vi "Begin.vi"   [LabVIEW 2012]
doc: "Called before other user functions, this VI is expected to open initial I/O refnums, load in file data, and do all program initialization. Notice that the <B>error out</B> terminal is simply used for data flow. Wiring it to other structures or subVIs ensures that this VI runs first."
uses:
  <vilib>/Rock Robotics/SystemInterfaces/Typedef/FPGA_TypedefDigitalModule.ctl
  <vilib>/Rock Robotics/SystemInterfaces/DIO/FPGA_DIOPWMChannel.ctl
  <vilib>/Rock Robotics/SystemInterfaces/DIO/FPGA_DIORelayChannel.ctl
  <vilib>/Rock Robotics/WPI/Relay/WPI_RelayDirection.ctl
  <vilib>/Rock Robotics/WPI/Joystick/WPI_JoystickDeviceEnum.ctl
  <vilib>/Rock Robotics/WPI/SafetyOutput/WPI_SafetyOutputConfigMenu.ctl
  <vilib>/Rock Robotics/WPI/MotorControl/WPI_MotorControlOpen Victor.vi
  <vilib>/Rock Robotics/WPI/MotorControl/WPI_MotorControlOpen Jaguar.vi
  <vilib>/Rock Robotics/WPI/RobotDrive/WPI_RobotDriveOpen4MotorWithJaguar.vi
  <vilib>/Rock Robotics/WPI/RobotDrive/WPI_RobotDriveOpen2MotorWithJaguar.vi
types:
  T1 = typedef "WPI_SafetyOutputConfigMenu.ctl" = enum16{"Enable", "Disable"}
  T2 = typedef "FPGA_DIOPWMChannel.ctl" = enum8{"PWM 1", "PWM 2", "PWM 3", "PWM 4", "PWM 5", "PWM 6", "PWM 7", "PWM 8", "PWM 9", "PWM 10", "Invalid"}
  T3 = typedef "WPI_RobotDriveDevRef.ctl" = cluster{"DevStatus":errorcluster, "Motors[]":T4[], "Square Inputs":bool, "Max Output":dbl, "Isochronous":bool}
  T4 = typedef "WPI_MotorControlDeviceRef.ctl" = cluster{"DeviceStatus":errorcluster, "Type":enum16{"PWM", "CAN"}, "PWM":cluster{"Digital Module":T5, "PWM Channel":T2, "DeadBand":T6}, "CAN":cluster{"Device Number":u8, "Control Mode":T7, "Semaphore":T8, "Max Vout":dbl}, "Invert":bool, "TransformRef":T9, "InvTransformRef":T9}
  T5 = typedef "FPGA_TypedefDigitalModule.ctl" = enum16{"Digital Module 1", "Digital Module 2"}
  T6 = typedef "WPI_PWMDeadband.ctl" = cluster{"Name":string, "maxPositivePwm":i32, "minPositivePwm":i32, "centerPwm":i32, "maxNegativePwm":i32, "minNegativePwm":i32, "angularRange":u16}
  T7 = typedef "WPI_CANJaguar_ControlMode.ctl" = enum8{"Percent VBus", "Current", "Speed", "Position", "Voltage"}
  T8 = typedef "Semaphore RefNum" = refnum<k1>
  T9 = typedef "WPI_PWMTransform_ConPane.ctl" = refnum<vi>
  T10 = typedef "WPI_RelayDirection.ctl" = enum16{"Both directions", "Forward only", "Reverse only"}
  T11 = typedef "FPGA_DIORelayChannel.ctl" = enum8{"Relay 1", "Relay 2", "Relay 3", "Relay 4", "Relay 5", "Relay 6", "Relay 7", "Relay 8", "Invalid"}
  T12 = typedef "WPI_ServoDeviceRef.ctl" = cluster{"DeviceStatus":errorcluster, "Digital Module":T5, "PWM Channel":T2, "DeadBand":T6}
  T13 = typedef "WPI_RelayDevRef.ctl" = cluster{"DevStatus":errorcluster, "Relay Channel":T11, "Digital Module":T5, "Relay Direction":T10}
  T14 = typedef "WPI_JoystickDeviceEnum.ctl" = enum16{"USB 1", "USB 2", "USB 3", "USB 4", "Kinect 1", "Kinect 2"}
  T15 = typedef "WPI_JoystickDevRef.ctl" = cluster{"Device":T14}
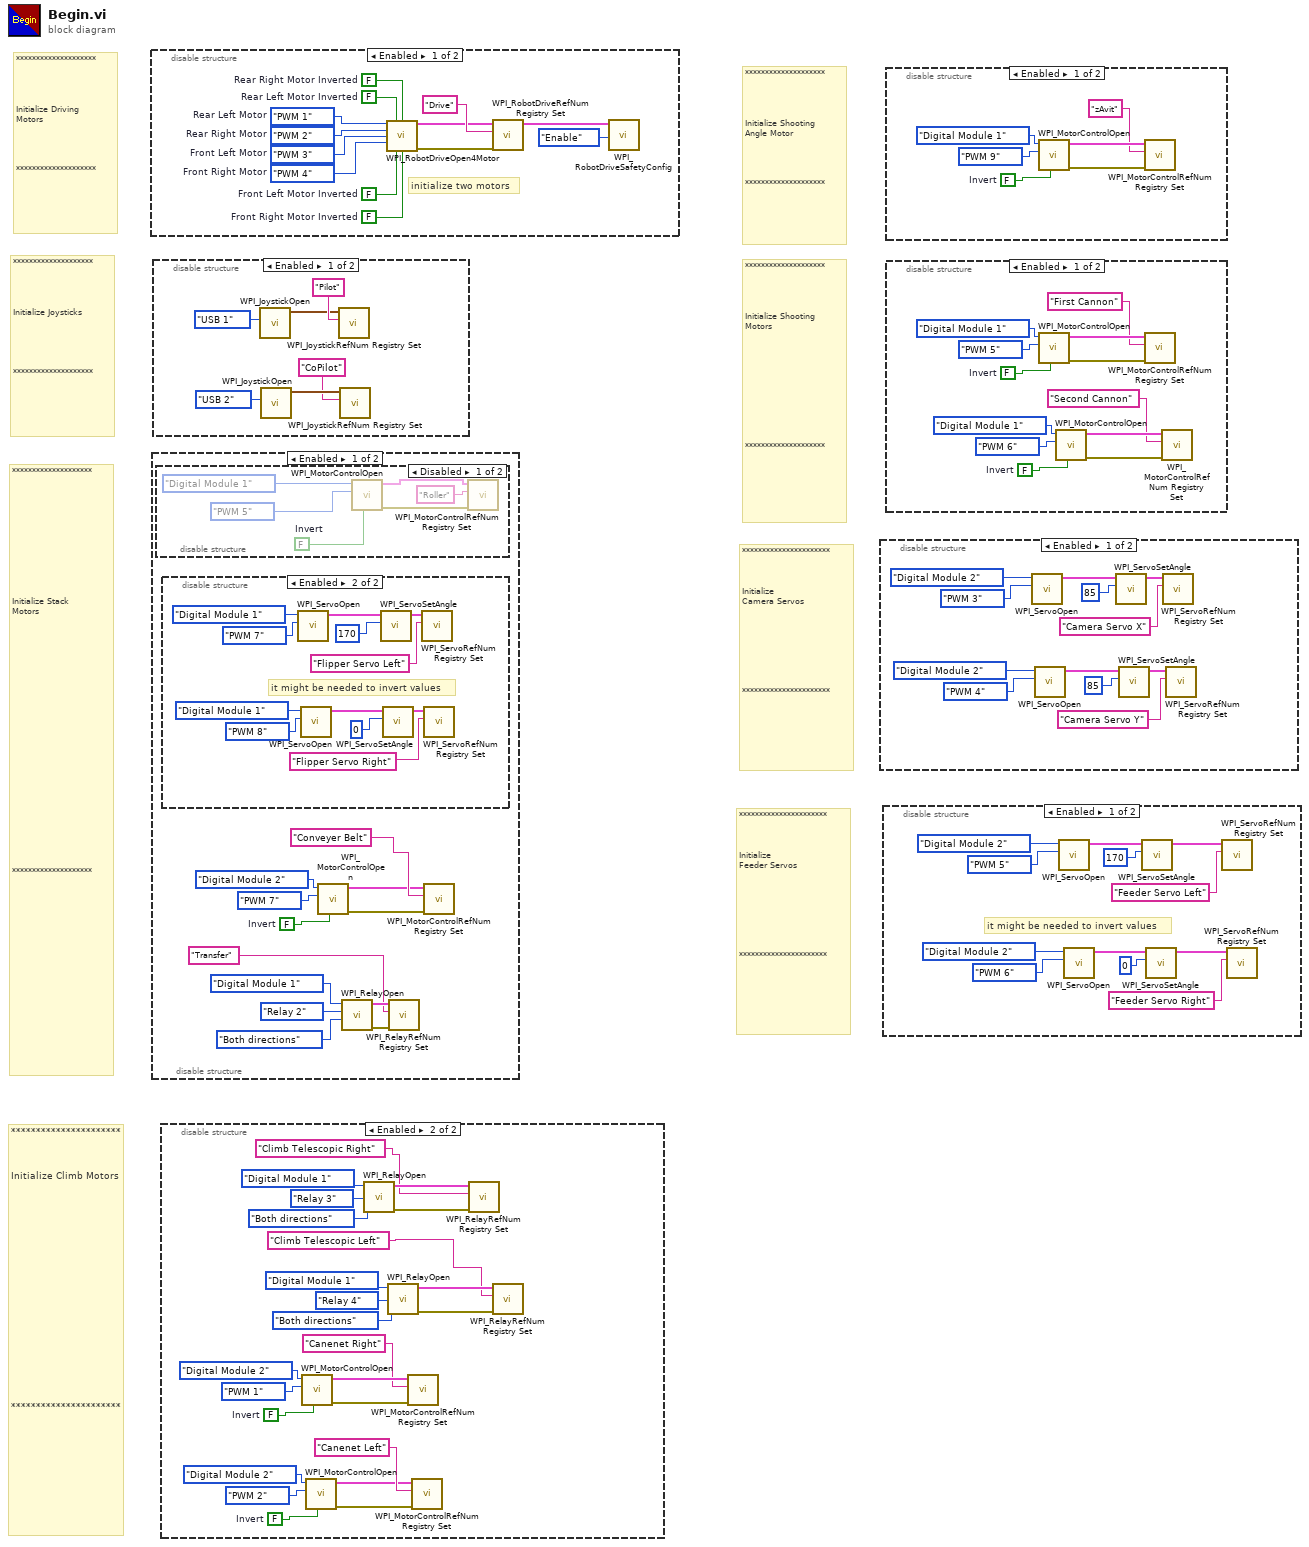
[diagram p0: block diagram]
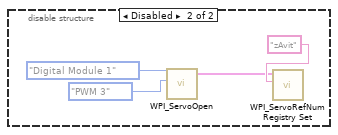
[diagram p5: hidden frame]
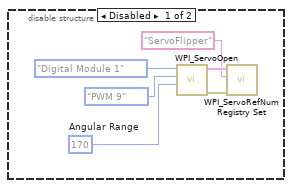
[diagram p9: hidden frame]
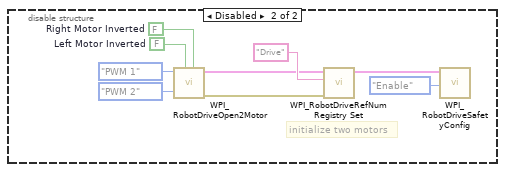
[diagram p11: hidden frame]
diagram:
  # "**********************\n\n\n\nInitialize\nFeeder Servos\n\n\n\n\n\n\n\n\n**********************"
  # "**********************\n\n\n\nInitialize\nCamera Servos\n\n\n\n\n\n\n\n\n**********************"
  # "**********************\n\n\n\nInitialize Climb Motors          \n\n\n\n\n\n\n\n\n\n\n\n\n\n\n\n\n\n\n\n\n**********************"
  # "********************\n\n\n\n\nInitialize Shooting\nAngle Motor\n\n\n\n\n********************"
  # "********************\n\n\n\n\nInitialize Shooting\nMotors\n\n\n\n\n\n\n\n\n\n\n\n********************"
  # "********************\n\n\n\n\n\n\n\n\n\n\n\n\nInitialize Stack \nMotors\n\n\n\n\n\n\n\n\n\n\n\n\n\n\n\n\n\n\n\n\n\n\n\n\n\n********************"
  # "********************\n\n\n\n\nInitialize Driving\nMotors\n\n\n\n\n********************"
  # "********************\n\n\n\n\nInitialize Joysticks\n\n\n\n\n\n********************"
  n1 = disable-structure shown="Enabled" {
    frame Enabled {
      w1 = FPGA_DIOPWMChannel."PWM 4"  # Front Right Motor
      w2 = FPGA_DIOPWMChannel."PWM 3"  # Front Left Motor
      w3 = FPGA_DIOPWMChannel."PWM 2"  # Rear Right Motor
      w4 = FPGA_DIOPWMChannel."PWM 1"  # Rear Left Motor
      w5 = FALSE  # Front Right Motor Inverted
      w6 = FALSE  # Front Left Motor Inverted
      w7 = FALSE  # Rear Right Motor Inverted
      w8 = FALSE  # Rear Left Motor Inverted
      # "initialize two motors"
      n2 = call-poly <vilib>:"WPI_RobotDriveOpen4Motor.vi"("Rear Left Motor"=w4, "Rear Left Motor Inverted"=w8, "Rear Right Motor Inverted"=w7, "Rear Right Motor"=w3, "Front Left Motor"=w2, "Front Right Motor"=w1, "Front Left Motor Inverted"=w6, "Front Right Motor Inverted"=w5) -> ("RobotDriveDevRef"=w10:T3, "error out"=w9:errorcluster)  [unwired: 6 in]
      n3 = call <vilib>:"WPI_RobotDriveRefNum Registry Set.vi"("error in (no error)"=w9, "refnum name"="Drive", "RobotDriveDevRef"=w10) -> ("RobotDriveDevRef"=w12:T3)  [unwired: 8 out]
      n4 = call <vilib>:"WPI_RobotDriveSafetyConfig.vi"("mode"=WPI_SafetyOutputConfigMenu."Enable", "RobotDriveDevRef"=w12) -> ()  [unwired: 8 in, 2 out]
    }
    frame Disabled {
      w14 = FALSE  # Right Motor Inverted
      w15 = FALSE  # Left Motor Inverted
      # "initialize two motors"
      n5 = call-poly <vilib>:"WPI_RobotDriveOpen2Motor.vi"("Right Motor Inverted"=w14, "Left Motor Inverted"=w15, "Right Motor"=FPGA_DIOPWMChannel."PWM 2", "Left Motor"=FPGA_DIOPWMChannel."PWM 1") -> ("error out"=w18:errorcluster, "RobotDriveDevRef"=w19:T3)  [unwired: 6 in]
      n6 = call <vilib>:"WPI_RobotDriveRefNum Registry Set.vi"("error in (no error)"=w18, "refnum name"="Drive", "RobotDriveDevRef"=w19) -> ("RobotDriveDevRef"=w21:T3)  [unwired: 8 out]
      n7 = call <vilib>:"WPI_RobotDriveSafetyConfig.vi"("mode"=WPI_SafetyOutputConfigMenu."Enable", "RobotDriveDevRef"=w21) -> ()  [unwired: 8 in, 2 out]
    }
  }
  n8 = disable-structure shown="Enabled" {
    frame Enabled {
      w24 = FALSE  # Invert
      n9 = disable-structure shown="Disabled" {
        frame Disabled {
          w36 = FALSE  # Invert
          n10 = call-poly <vilib>:"WPI_MotorControlOpen.vi"("Invert"=w36, "PWM Channel"=FPGA_DIOPWMChannel."PWM 5", "Digital Module (Module 1)"=FPGA_TypedefDigitalModule."Digital Module 1") -> ("error out"=w35:errorcluster, "MotorControlDeviceRef"=w40:T4)  [unwired: 7 in]
          n11 = call <vilib>:"WPI_MotorControlRefNum Registry Set.vi"("error in (no error)"=w35, "refnum name"="Roller", "MotorControlDevRef"=w40) -> ()  [unwired: 7 in, 2 out]
        }
        frame Enabled {
        }
      }
      n12 = disable-structure shown="Enabled" {
        frame Disabled {
          w43 = u16 170  # Angular Range
          n13 = call <vilib>:"WPI_ServoOpen.vi"("Angular Range"=w43, "PWM Channel"=FPGA_DIOPWMChannel."PWM 9", "Digital Module (Module 1)"=FPGA_TypedefDigitalModule."Digital Module 1") -> ("error out"=w42:errorcluster, "ServoDeviceRef"=w46:T12)  [unwired: 7 in]
          n14 = call <vilib>:"WPI_ServoRefNum Registry Set.vi"("error in (no error)"=w42, "refnum name"="ServoFlipper", "ServoDeviceRef"=w46) -> ()  [unwired: 7 in, 2 out]
        }
        frame Enabled {
          # "it might be needed to invert values"
          n15 = call <vilib>:"WPI_ServoOpen.vi"("PWM Channel"=FPGA_DIOPWMChannel."PWM 7", "Digital Module (Module 1)"=FPGA_TypedefDigitalModule."Digital Module 1") -> ("ServoDeviceRef"=w58:T12)  [unwired: 8 in, 1 out]
          n16 = call <vilib>:"WPI_ServoOpen.vi"("PWM Channel"=FPGA_DIOPWMChannel."PWM 8", "Digital Module (Module 1)"=FPGA_TypedefDigitalModule."Digital Module 1") -> ("ServoDeviceRef"=w48:T12)  [unwired: 8 in, 1 out]
          n17 = call <vilib>:"WPI_ServoSetAngle.vi"("Angle"=170, "ServoDeviceRef"=w58) -> ("ServoDeviceRef"=w54:T12)  [unwired: 8 in, 1 out]
          n18 = call <vilib>:"WPI_ServoSetAngle.vi"("Angle"=0, "ServoDeviceRef"=w48) -> ("ServoDeviceRef"=w51:T12)  [unwired: 8 in, 1 out]
          n19 = call <vilib>:"WPI_ServoRefNum Registry Set.vi"("refnum name"="Flipper Servo Left", "ServoDeviceRef"=w54) -> ()  [unwired: 8 in, 2 out]
          n20 = call <vilib>:"WPI_ServoRefNum Registry Set.vi"("refnum name"="Flipper Servo Right", "ServoDeviceRef"=w51) -> ()  [unwired: 8 in, 2 out]
        }
      }
      n21 = call-poly <vilib>:"WPI_MotorControlOpen.vi"("Invert"=w24, "PWM Channel"=FPGA_DIOPWMChannel."PWM 7", "Digital Module (Module 1)"=FPGA_TypedefDigitalModule."Digital Module 2") -> ("error out"=w23:errorcluster, "MotorControlDeviceRef"=w27:T4)  [unwired: 7 in]
      n22 = call <vilib>:"WPI_RelayOpen.vi"("Relay Direction"=WPI_RelayDirection."Both directions", "Relay Channel"=FPGA_DIORelayChannel."Relay 2", "Digital Module (Module 1)"=FPGA_TypedefDigitalModule."Digital Module 1") -> ("error out"=w31:errorcluster, "RelayDevRef"=w30:T13)  [unwired: 7 in]
      n23 = call <vilib>:"WPI_RelayRefNum Registry Set.vi"("error in (no error)"=w31, "refnum name"="Transfer", "RelayDevRef"=w30) -> ()  [unwired: 7 in, 2 out]
      n24 = call <vilib>:"WPI_MotorControlRefNum Registry Set.vi"("error in (no error)"=w23, "refnum name"="Conveyer Belt", "MotorControlDevRef"=w27) -> ()  [unwired: 7 in, 2 out]
    }
    frame Disabled {
    }
  }
  n25 = disable-structure shown="Enabled" {
    frame Enabled {
      n26 = call <vilib>:"WPI_JoystickOpen.vi"("JoystickDevice"=WPI_JoystickDeviceEnum."USB 1") -> ("JoystickDevRef"=w63:T15)  [unwired: 10 in]
      n27 = call <vilib>:"WPI_JoystickOpen.vi"("JoystickDevice"=WPI_JoystickDeviceEnum."USB 2") -> ("JoystickDevRef"=w60:T15)  [unwired: 10 in]
      n28 = call <vilib>:"WPI_JoystickRefNum Registry Set.vi"("refnum name"="Pilot", "JoystickDevRef"=w63) -> ()  [unwired: 8 in, 2 out]
      n29 = call <vilib>:"WPI_JoystickRefNum Registry Set.vi"("refnum name"="CoPilot", "JoystickDevRef"=w60) -> ()  [unwired: 8 in, 2 out]
    }
    frame Disabled {
    }
  }
  n30 = disable-structure shown="Enabled" {
    frame Disabled {
    }
    frame Enabled {
      w81 = FALSE  # Invert
      w84 = FALSE  # Invert
      n31 = call-poly <vilib>:"WPI_MotorControlOpen.vi"("Invert"=w84, "PWM Channel"=FPGA_DIOPWMChannel."PWM 1", "Digital Module (Module 1)"=FPGA_TypedefDigitalModule."Digital Module 2") -> ("error out"=w83:errorcluster, "MotorControlDeviceRef"=w88:T4)  [unwired: 7 in]
      n32 = call-poly <vilib>:"WPI_MotorControlOpen.vi"("Invert"=w81, "PWM Channel"=FPGA_DIOPWMChannel."PWM 2", "Digital Module (Module 1)"=FPGA_TypedefDigitalModule."Digital Module 2") -> ("error out"=w82:errorcluster, "MotorControlDeviceRef"=w77:T4)  [unwired: 7 in]
      n33 = call <vilib>:"WPI_RelayOpen.vi"("Relay Direction"=WPI_RelayDirection."Both directions", "Relay Channel"=FPGA_DIORelayChannel."Relay 3", "Digital Module (Module 1)"=FPGA_TypedefDigitalModule."Digital Module 1") -> ("error out"=w75:errorcluster, "RelayDevRef"=w76:T13)  [unwired: 7 in]
      n34 = call <vilib>:"WPI_RelayOpen.vi"("Relay Direction"=WPI_RelayDirection."Both directions", "Relay Channel"=FPGA_DIORelayChannel."Relay 4", "Digital Module (Module 1)"=FPGA_TypedefDigitalModule."Digital Module 1") -> ("error out"=w69:errorcluster, "RelayDevRef"=w70:T13)  [unwired: 7 in]
      n35 = call <vilib>:"WPI_MotorControlRefNum Registry Set.vi"("error in (no error)"=w83, "refnum name"="Canenet Right", "MotorControlDevRef"=w88) -> ()  [unwired: 7 in, 2 out]
      n36 = call <vilib>:"WPI_MotorControlRefNum Registry Set.vi"("error in (no error)"=w82, "refnum name"="Canenet Left", "MotorControlDevRef"=w77) -> ()  [unwired: 7 in, 2 out]
      n37 = call <vilib>:"WPI_RelayRefNum Registry Set.vi"("error in (no error)"=w75, "refnum name"="Climb Telescopic Right", "RelayDevRef"=w76) -> ()  [unwired: 7 in, 2 out]
      n38 = call <vilib>:"WPI_RelayRefNum Registry Set.vi"("error in (no error)"=w69, "refnum name"="Climb Telescopic Left", "RelayDevRef"=w70) -> ()  [unwired: 7 in, 2 out]
    }
  }
  n39 = disable-structure shown="Enabled" {
    frame Enabled {
      n40 = call <vilib>:"WPI_ServoOpen.vi"("PWM Channel"=FPGA_DIOPWMChannel."PWM 3", "Digital Module (Module 1)"=FPGA_TypedefDigitalModule."Digital Module 2") -> ("ServoDeviceRef"=w97:T12)  [unwired: 8 in, 1 out]
      n41 = call <vilib>:"WPI_ServoOpen.vi"("PWM Channel"=FPGA_DIOPWMChannel."PWM 4", "Digital Module (Module 1)"=FPGA_TypedefDigitalModule."Digital Module 2") -> ("ServoDeviceRef"=w92:T12)  [unwired: 8 in, 1 out]
      n42 = call <vilib>:"WPI_ServoSetAngle.vi"("Angle"=85, "ServoDeviceRef"=w97) -> ("ServoDeviceRef"=w96:T12)  [unwired: 8 in, 1 out]
      n43 = call <vilib>:"WPI_ServoSetAngle.vi"("Angle"=85, "ServoDeviceRef"=w92) -> ("ServoDeviceRef"=w93:T12)  [unwired: 8 in, 1 out]
      n44 = call <vilib>:"WPI_ServoRefNum Registry Set.vi"("refnum name"="Camera Servo X", "ServoDeviceRef"=w96) -> ()  [unwired: 8 in, 2 out]
      n45 = call <vilib>:"WPI_ServoRefNum Registry Set.vi"("refnum name"="Camera Servo Y", "ServoDeviceRef"=w93) -> ()  [unwired: 8 in, 2 out]
    }
    frame Disabled {
    }
  }
  n46 = disable-structure shown="Enabled" {
    frame Enabled {
      # "it might be needed to invert values"
      n47 = call <vilib>:"WPI_ServoOpen.vi"("PWM Channel"=FPGA_DIOPWMChannel."PWM 5", "Digital Module (Module 1)"=FPGA_TypedefDigitalModule."Digital Module 2") -> ("ServoDeviceRef"=w109:T12)  [unwired: 8 in, 1 out]
      n48 = call <vilib>:"WPI_ServoOpen.vi"("PWM Channel"=FPGA_DIOPWMChannel."PWM 6", "Digital Module (Module 1)"=FPGA_TypedefDigitalModule."Digital Module 2") -> ("ServoDeviceRef"=w108:T12)  [unwired: 8 in, 1 out]
      n49 = call <vilib>:"WPI_ServoSetAngle.vi"("Angle"=170, "ServoDeviceRef"=w109) -> ("ServoDeviceRef"=w104:T12)  [unwired: 8 in, 1 out]
      n50 = call <vilib>:"WPI_ServoSetAngle.vi"("Angle"=0, "ServoDeviceRef"=w108) -> ("ServoDeviceRef"=w103:T12)  [unwired: 8 in, 1 out]
      n51 = call <vilib>:"WPI_ServoRefNum Registry Set.vi"("refnum name"="Feeder Servo Left", "ServoDeviceRef"=w104) -> ()  [unwired: 8 in, 2 out]
      n52 = call <vilib>:"WPI_ServoRefNum Registry Set.vi"("refnum name"="Feeder Servo Right", "ServoDeviceRef"=w103) -> ()  [unwired: 8 in, 2 out]
    }
    frame Disabled {
    }
  }
  n53 = disable-structure shown="Enabled" {
    frame Enabled {
      w114 = FALSE  # Invert
      n54 = call-poly <vilib>:"WPI_MotorControlOpen.vi"("Invert"=w114, "PWM Channel"=FPGA_DIOPWMChannel."PWM 9", "Digital Module (Module 1)"=FPGA_TypedefDigitalModule."Digital Module 1") -> ("error out"=w113:errorcluster, "MotorControlDeviceRef"=w118:T4)  [unwired: 7 in]
      n55 = call <vilib>:"WPI_MotorControlRefNum Registry Set.vi"("error in (no error)"=w113, "refnum name"="zAvit", "MotorControlDevRef"=w118) -> ()  [unwired: 7 in, 2 out]
    }
    frame Disabled {
      n56 = call <vilib>:"WPI_ServoOpen.vi"("PWM Channel"=FPGA_DIOPWMChannel."PWM 3", "Digital Module (Module 1)"=FPGA_TypedefDigitalModule."Digital Module 1") -> ("ServoDeviceRef"=w119:T12)  [unwired: 8 in, 1 out]
      n57 = call <vilib>:"WPI_ServoRefNum Registry Set.vi"("refnum name"="zAvit", "ServoDeviceRef"=w119) -> ()  [unwired: 8 in, 2 out]
    }
  }
  n58 = disable-structure shown="Enabled" {
    frame Enabled {
      w124 = FALSE  # Invert
      w130 = FALSE  # Invert
      n59 = call-poly <vilib>:"WPI_MotorControlOpen.vi"("Invert"=w130, "PWM Channel"=FPGA_DIOPWMChannel."PWM 5", "Digital Module (Module 1)"=FPGA_TypedefDigitalModule."Digital Module 1") -> ("error out"=w129:errorcluster, "MotorControlDeviceRef"=w134:T4)  [unwired: 7 in]
      n60 = call-poly <vilib>:"WPI_MotorControlOpen.vi"("Invert"=w124, "PWM Channel"=FPGA_DIOPWMChannel."PWM 6", "Digital Module (Module 1)"=FPGA_TypedefDigitalModule."Digital Module 1") -> ("error out"=w123:errorcluster, "MotorControlDeviceRef"=w128:T4)  [unwired: 7 in]
      n61 = call <vilib>:"WPI_MotorControlRefNum Registry Set.vi"("error in (no error)"=w129, "refnum name"="First Cannon", "MotorControlDevRef"=w134) -> ()  [unwired: 7 in, 2 out]
      n62 = call <vilib>:"WPI_MotorControlRefNum Registry Set.vi"("error in (no error)"=w123, "refnum name"="Second Cannon", "MotorControlDevRef"=w128) -> ()  [unwired: 7 in, 2 out]
    }
    frame Disabled {
    }
  }
